vi "Read Humidity Cal.vi"(8 "error in (no error)":errorcluster, 11 "LINX I2C in":refnum<class "LINX I2C.lvclass">) -> (0 "error out":errorcluster, 1 "Zero":dbl, 2 "Slope":dbl, 3 "LINX I2C out":refnum<class "LINX I2C.lvclass">)   [LabVIEW 2020, in "HTS221.lvclass"]
uses:
  HTS221.lvclass
  LINX I2C/LINX I2C.lvclass
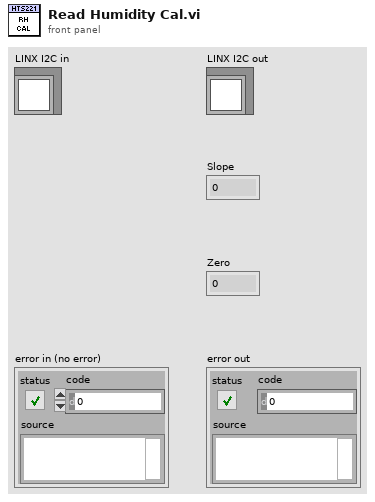
[diagram p1: front panel]
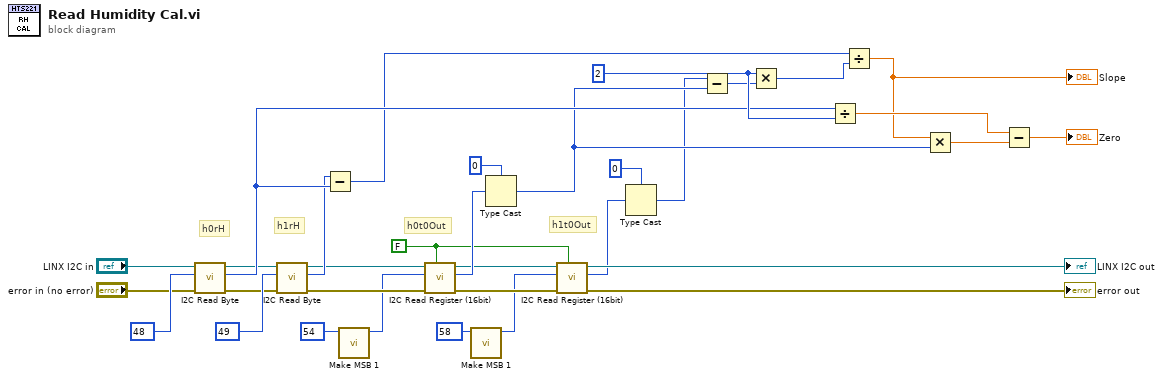
[diagram p0: block diagram]
diagram:
  w1 = FALSE ("MSB(yte) First? (T)")
  w31 = i16 2 ("x")
  # "h1t0Out"
  # "h0t0Out"
  # "h1rH"
  # "h0rH"
  n1 = call-dynamic "I2C Read Byte.vi"("error in (no error)"="error in (no error)", "Register Address"=u8 48, "LINX I2C in"="LINX I2C in") -> ("error out"=w8:errorcluster, "Byte Read"=w26:u8, "LINX I2C out"=w7:refnum<class "LINX I2C.lvclass">)  [unwired: 6 in]
  n2 = call-dynamic "I2C Read Byte.vi"("error in (no error)"=w8, "Register Address"=u8 49, "LINX I2C in"=w7) -> ("error out"=w11:errorcluster, "Byte Read"=w18:u8, "LINX I2C out"=w10:refnum<class "LINX I2C.lvclass">)  [unwired: 6 in]
  n3 = Subtract(x=w18, y=w26) -> (x-y=w19:u8)
  n4 = call "Make MSB 1.vi"("Register Address"=u8 54) -> ("Register Address | 0x80"=w4:u8)  [unwired: 10 in]
  n5 = call "I2C Read Register (16bit).vi"("MSB(yte) First? (F=Lo->Hi)"=w1, "error in (no error)"=w11, "Register Address"=w4, "LINX I2C in"=w10) -> ("error out"=w13:errorcluster, "Value"=w17:u16, "LINX I2C out"=w12:refnum<class "LINX I2C.lvclass">)  [unwired: 5 in]
  n6 = call "Make MSB 1.vi"("Register Address"=u8 58) -> ("Register Address | 0x80"=w2:u8)  [unwired: 10 in]
  n7 = Type Cast(type=i16 0, x=w17) -> (*(type *) &x=w24:i16)
  n8 = call "I2C Read Register (16bit).vi"("MSB(yte) First? (F=Lo->Hi)"=w1, "error in (no error)"=w13, "Register Address"=w2, "LINX I2C in"=w12) -> ("error out"=→"error out":errorcluster, "Value"=w14:u16, "LINX I2C out"=→"LINX I2C out":refnum<class "LINX I2C.lvclass">)  [unwired: 5 in]
  n9 = Type Cast(type=i16 0, x=w14) -> (*(type *) &x=w20:i16)
  n10 = Subtract(x=w20, y=w24) -> (x-y=w21:i16)
  n11 = Multiply(x=w31, y=w21) -> (x*y=w22:i16)
  n12 = Divide(x=w26, y=w31) -> (x/y=w27:dbl)
  n13 = Divide(x=w19, y=w22) -> (x/y=w23:dbl)
  "Slope" <- w23
  n14 = Multiply(x=w23, y=w24) -> (x*y=w25:dbl)
  n15 = Subtract(x=w27, y=w25) -> (x-y=→"Zero":dbl)
